vi "config.vi"() -> ()   [LabVIEW 2015]
uses:
  board.vis/Globals.vi
  board.vis/ESLSCDLL.lvlib
panel:
  in  "DLL path select":enum32{"default location", "custom location"}(radio)
  in  "DLL custom path":path
  in  "shift S1S2 to next scan":bool
  in  "channel select":enum32{"Channel A", "Channel B", "Channel A&B"}(ring)=enum."Channel A&B"
  in  "show shutter":bool
  in  "bticnt":u32
  in  "is fft legacy":bool
  in  "s1s2_read_delay_in_10ns":u32
  in  "bnc_out":T1(ring)
  in  "sensor reset or HSIR EC":u32
  in  "SENSOR TYPE":T2(ring)=enum."HSVIS"
  in  "dac":u32[][][](array[numeric])=[[[55000, 52000, 55000, 55000, 55000, 55000, 55000, 55000], [55000, 52000, 55000, 55000, 55000, 55000, 55000, 55000], [55000, 52000, 55000, 55000, 55000, 55000, 55000, 55000], [55000, 52000, 55000, 55000, 55000, 55000, 55000, 55000], [55000, 52000, 55000, 55000, 55000, 55000, 55000, 55000], [55000, 52000, 55000, 55000, 55000, 55000, 55000, 55000], [55000, 52000, 55000, 55000, 55000, 55000, 55000, 55000], [55000, 52000, 55000, 55001, 55000, 55000, 55000, 55000], [55000, 55000, 55000, 55000, 55000, 55000, 55000, 55000], [55000, 55000, 55000, 55000, 55000, 55000, 55000, 55000], [55000, 55000, 55000, 55000, 55000, 55000, 55000, 55000], [55000, 55000, 55000, 55000, 55000, 55000, 55000, 55000]], [[52000, 0, 0, 0, 0, 0, 0, 0], [52000, 0, 0, 0, 0, 0, 0, 0], [52000, 0, 0, 0, 0, 0, 0, 0], [52000, 0, 0, 0, 0, 0, 0, 0], [52000, 0, 0, 0, 0, 0, 0, 0], [52000, 0, 0, 0, 0, 0, 0, 0], [52000, 0, 0, 0, 0, 0, 0, 0], [52000, 0, 0, 0, 0, 0, 0, 0], [0, 0, 0, 0, 0, 0, 0, 0], [0, 0, 0, 0, 0, 0, 0, 0], [0, 0, 0, 0, 0, 0, 0, 0], [0, 0, 0, 0, 0, 0, 0, 0]], [[52000, 0, 0, 0, 0, 0, 0, 0], [52000, 0, 0, 0, 0, 0, 0, 0], [52000, 0, 0, 0, 0, 0, 0, 0], [52000, 0, 0, 0, 0, 0, 0, 0], [52000, 0, 0, 0, 0, 0, 0, 0], [52000, 0, 0, 0, 0, 0, 0, 0], [52000, 0, 0, 0, 0, 0, 0, 0], [52000, 0, 0, 0, 0, 0, 0, 0], [0, 0, 0, 0, 0, 0, 0, 0], [0, 0, 0, 0, 0, 0, 0, 0], [0, 0, 0, 0, 0, 0, 0, 0], [0, 0, 0, 0, 0, 0, 0, 0]], [[52000, 0, 0, 0, 0, 0, 0, 0], [52000, 0, 0, 0, 0, 0, 0, 0], [52000, 0, 0, 0, 0, 0, 0, 0], [52000, 0, 0, 0, 0, 0, 0, 0], [52000, 0, 0, 0, 0, 0, 0, 0], [52000, 0, 0, 0, 0, 0, 0, 0], [52000, 0, 0, 0, 0, 0, 0, 0], [52000, 0, 0, 0, 0, 0, 0, 0], [0, 0, 0, 0, 0, 0, 0, 0], [0, 0, 0, 0, 0, 0, 0, 0], [0, 0, 0, 0, 0, 0, 0, 0], [0, 0, 0, 0, 0, 0, 0, 0]], [[52000, 0, 0, 0, 0, 0, 0, 0], [52000, 0, 0, 0, 0, 0, 0, 0], [52000, 0, 0, 0, 0, 0, 0, 0], [52000, 0, 0, 0, 0, 0, 0, 0], [52000, 0, 0, 0, 0, 0, 0, 0], [52000, 0, 0, 0, 0, 0, 0, 0], [52000, 0, 0, 0, 0, 0, 0, 0], [52000, 0, 0, 0, 0, 0, 0, 0], [0, 0, 0, 0, 0, 0, 0, 0], [0, 0, 0, 0, 0, 0, 0, 0], [0, 0, 0, 0, 0, 0, 0, 0], [0, 0, 0, 0, 0, 0, 0, 0]]]
  in  "stime[ms]":dbl=0.01 format="%-3.3f"
  in  "btime[ms]":dbl=31.0 format="%1.3f"
  in  "sdat in 10ns":u32
  in  "bdat in 10ns":u32
  in  "bti":T3(ring)=enum."BTimer"
  in  "sti":T4(ring)=enum."STimer"
  in  "trigger mode integrator":enum32{"XCK", "Ext. Trig.", "DAT"}(ring)
  in  "bt slope":enum32{"neg", "pos", "both"}(ring)=enum."pos"
  in  "st slope":enum32{"pos", "neg", "both"}(ring)
  in  "custom pattern":u32=100
  in  "adc mode":enum32{"normal", "ramp", "custom pattern"}(ring)
  in  "fft mode":T5(ring)
  in  "cool level":u32
  in  "board_sel":u32=1 format="%05b"
  in  "sticnt":u32
  in  "show pulse gen":bool
  in  "show special pixels":bool
  in  "debug mode":bool
  in  "show one pixel graph":bool
  in  "adc gain":u32
  in  "area lines binning":u32=1
  in  "nor":u32=3
  in  "region size":u32[](array[numeric])=[4, 62, 4, 28, 14, 0, 0, 0]
  in  "LINES":u32=128
  in  "VFREQ":u32=7
  in  "software polling":bool
  in  "led off":bool
  in  "tocnt":u32
  in  "ioctrl impact start pixel":u32=1050
  in  "cont pause in microseconds":u32
  in  "tor":T6(ring)
  in  "write to disc":bool
  in  "file path":path
  in  "cooled camera legacy mode":bool
  in  "cooled cam":bool
  in  "sensor gain":u32
  in  "gpx offset":u32=1000
  in  "xckdly in 10ns (legacy)":u32
  in  "bec in 10\nns":u32
  in  "sec in 10ns":u32
  in  "CAMCNT 4":u32=1
  in  "CAMCNT 3":u32=1
  in  "CAMCNT 2":u32=1
  in  "CAMCNT 1":u32=1
  in  "CAMCNT 0":u32=1
  in  "CAMERA SYSTEM":enum32{"3001", "3010", "3030"}(ring)=enum."3030"
  in  "PIXEL":u32=1024
  # "camera system settings"
  # "measurement settings"
  # "Pixel sizes:\n192\n320\n576\n1024(HSVIS)\n1088\n2112\n4160\n8256"
  # "output PCIe board"
  # "scan exposue control"
  # "pause for continuous mode in µs"
  # "block exposure control"
  # "block delay after trigger"
  # "CAMCNT\nnumber of \ncameras per board"
  # "only for TDC option"
  # "depending on SENSOR TYPE\nthe actual time is\nHSVIS: time = x * 4 ns\nHSIR: time = x * 160 ns"
  # "fft setttings"
  # "only for FL30XX_simple.vi"
  # "labview"
  # "Select boards bitwise. Bit 0 - board 0 ....\nFor one board: 00001"
  # "lines of camera"
  # "Choose how many lines are binned in area mode.\nare_lines_binning should devide lines without remainder"
  # "number of regions for regions of interest mode\n(choose from 2 to 5)"
  # "count of lines for each region.\nWhen 0 is selected for the first region,\nthe lines are equally distributed over all regions.\nWhen selecting custom values,\nthe sum of all regions should equal lines."
  # "High Speed, 3030"
  # "camera 4"
  # "camera 6"
  # "camera 7"
  # "camera 0"
  # "camera 1"
  # "camera 3"
  # "camera 5"
  # "camera 2"
  # "PCIe board (0 ... 4) -->"
  # "channel 0"
  # "keep 0 -->"
  # "channel 1"
  # "keep 0 -->"
  # "channel 2"
  # "channel 3"
  # "channel 4"
  # "channel 5"
  # "channel 6"
  # "channel 7"
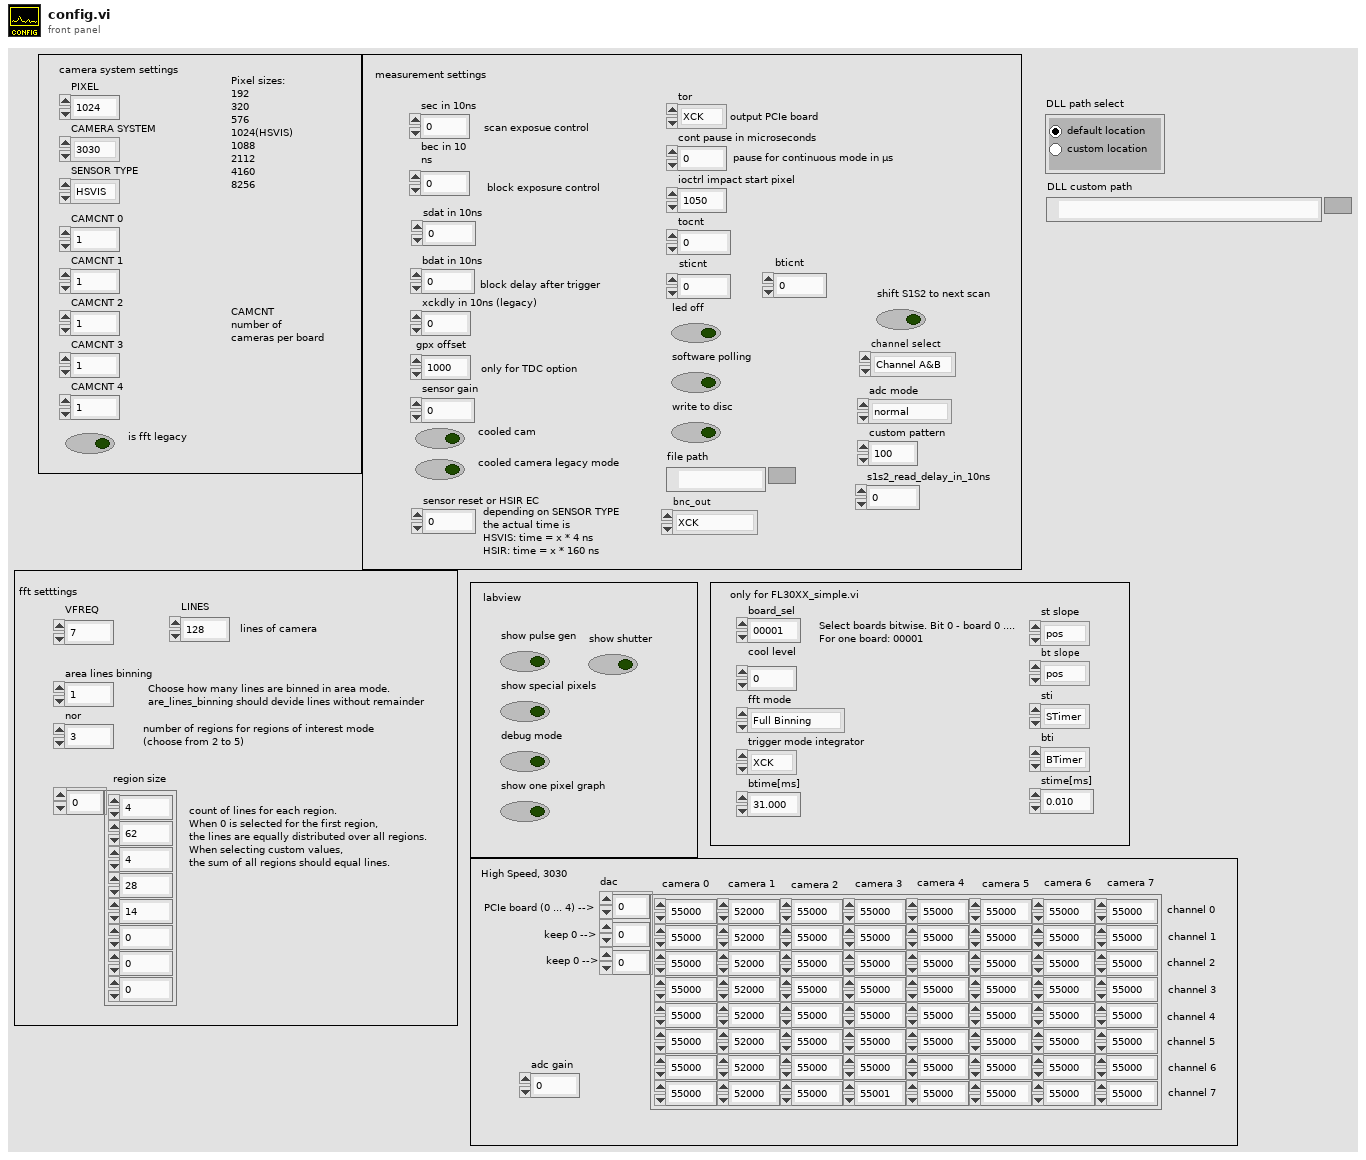
[diagram p1: front panel]
types:
  T1 = enum32{"XCK", "EXP_WIN", "ADC_CLK", "Vin sample"}
  T2 = enum32{"PDA", "IR", "FFT", "CMOS", "HSVIS", "HSIR"}
  T3 = enum32{"I", "S1", "S2", "S1&S2", "BTimer", "S1 chopper", "S2 chopper", "S1&S2 chopper"}
  T4 = enum32{"I", "S1", "S2", "S2=EN_I", "STimer", "ASL"}
  T5 = enum32{"Full Binning", "Region of Interest", "Area"}
  T6 = enum32{"XCK", "Reg/OutTrig", "VON", "DMA_Act", "ASLS", "STIMER", "BTIMER", "INTRSR", "S1", "S2", "BLOCK_ON_SYNCED", "MEASUREON", "SDAT", "BDAT", "SSHUT", "BSHUT", "IFC", "DO_CC_I", "EXPOSURE_WINDOW", "TO_CNT_OUT", "SECON", "I", "S1S2ReadDelay", "BLOCK_ON", "unused4", "unused5", "unused6", "unused7", "unused8", "ENFFR", "ENFFW", "ENFFWRPROT"}
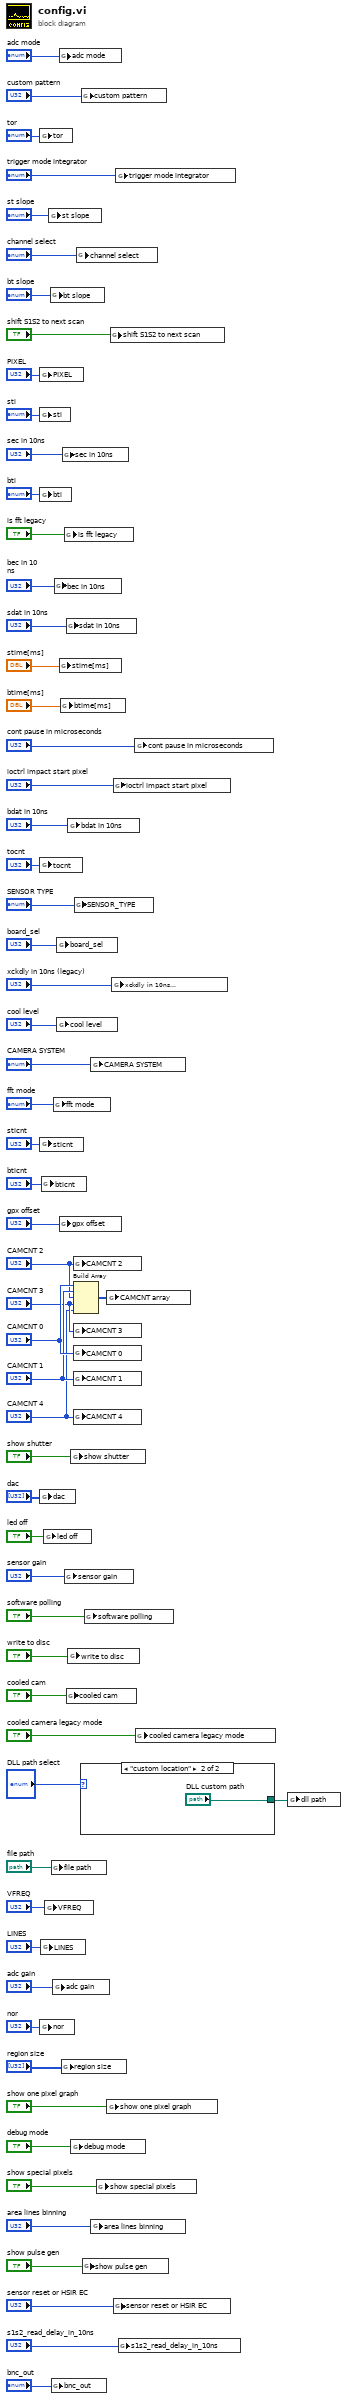
[diagram p0: block diagram]
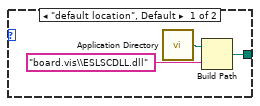
[diagram p2: hidden frame]
diagram:
  n1 = global write "Globals.vi" "tor"("tor") -> ()
  n2 = global write "Globals.vi" "PIXEL"("PIXEL") -> ()
  n3 = global write "Globals.vi" "sti"("sti") -> ()
  n4 = global write "Globals.vi" "bti"("bti") -> ()
  n5 = global write "Globals.vi" "tocnt"("tocnt") -> ()
  n6 = global write "Globals.vi" "sticnt"("sticnt") -> ()
  n7 = global write "Globals.vi" "dac"("dac") -> ()
  n8 = global write "Globals.vi" "nor"("nor") -> ()
  n9 = global write "Globals.vi" "LINES"("LINES") -> ()
  n10 = global write "Globals.vi" "bticnt"("bticnt") -> ()
  n11 = global write "Globals.vi" "led off"("led off") -> ()
  n12 = global write "Globals.vi" "VFREQ"("VFREQ") -> ()
  n13 = global write "Globals.vi" "st slope"("st slope") -> ()
  n14 = global write "Globals.vi" "bt slope"("bt slope") -> ()
  n15 = global write "Globals.vi" "file path"("file path") -> ()
  n16 = global write "Globals.vi" "bnc_out"("bnc_out") -> ()
  n17 = global write "Globals.vi" "adc gain"("adc gain") -> ()
  n18 = global write "Globals.vi" "fft mode"("fft mode") -> ()
  n19 = global write "Globals.vi" "bec in 10ns"("bec in 10\nns") -> ()
  n20 = global write "Globals.vi" "board_sel"("board_sel") -> ()
  n21 = global write "Globals.vi" "cool level"("cool level") -> ()
  n22 = global write "Globals.vi" "adc mode"("adc mode") -> ()
  n23 = global write "Globals.vi" "stime[ms]"("stime[ms]") -> ()
  n24 = global write "Globals.vi" "gpx offset"("gpx offset") -> ()
  n25 = global write "Globals.vi" "btime[ms]"("btime[ms]") -> ()
  n26 = global write "Globals.vi" "region size"("region size") -> ()
  n27 = global write "Globals.vi" "sec in 10ns"("sec in 10ns") -> ()
  n28 = global write "Globals.vi" "is fft legacy"("is fft legacy") -> ()
  n29 = global write "Globals.vi" "sensor gain"("sensor gain") -> ()
  n30 = global write "Globals.vi" "sdat in 10ns"("sdat in 10ns") -> ()
  n31 = global write "Globals.vi" "cooled cam"("cooled cam") -> ()
  n32 = global write "Globals.vi" "bdat in 10ns"("bdat in 10ns") -> ()
  n33 = global write "Globals.vi" "write to disc"("write to disc") -> ()
  n34 = global write "Globals.vi" "show shutter"("show shutter") -> ()
  n35 = global write "Globals.vi" "debug mode"("debug mode") -> ()
  n36 = global write "Globals.vi" "CAMCNT 2"("CAMCNT 2") -> ()
  n37 = Build Array("CAMCNT 0", "CAMCNT 1", "CAMCNT 2", "CAMCNT 3", "CAMCNT 4") -> (w55:u32[])
  n38 = global write "Globals.vi" "CAMCNT 3"("CAMCNT 3") -> ()
  n39 = global write "Globals.vi" "CAMCNT 0"("CAMCNT 0") -> ()
  n40 = global write "Globals.vi" "CAMCNT 1"("CAMCNT 1") -> ()
  n41 = global write "Globals.vi" "CAMCNT 4"("CAMCNT 4") -> ()
  n42 = global write "Globals.vi" "SENSOR_TYPE"("SENSOR TYPE") -> ()
  n43 = global write "Globals.vi" "channel select"("channel select") -> ()
  n44 = case shown="\"custom location\"" "DLL path select" {
    tunnel: [w61 "DLL custom path"] -> w1
    frame "default location", Default {
      n45 = call <vilib>:"Application Directory.vi"() -> ("Application Directory"=w62:path)
      n46 = Build Path(base path=w62, name or relative path="board.vis\\ESLSCDLL.dll") -> (appended path=w61:path)
    }
    frame "custom location" {
    }
  }
  n47 = global write "Globals.vi" "custom pattern"("custom pattern") -> ()
  n48 = global write "Globals.vi" "show pulse gen"("show pulse gen") -> ()
  n49 = global write "Globals.vi" "software polling"("software polling") -> ()
  n50 = global write "Globals.vi" "CAMERA SYSTEM"("CAMERA SYSTEM") -> ()
  n51 = global write "Globals.vi" "area lines binning"("area lines binning") -> ()
  n52 = global write "Globals.vi" "show special pixels"("show special pixels") -> ()
  n53 = global write "Globals.vi" "CAMCNT array"(w55) -> ()
  n54 = global write "Globals.vi" "show one pixel graph"("show one pixel graph") -> ()
  n55 = global write "Globals.vi" "shift S1S2 to next scan"("shift S1S2 to next scan") -> ()
  n56 = global write "Globals.vi" "xckdly in 10ns\n(legacy)"("xckdly in 10ns (legacy)") -> ()
  n57 = global write "Globals.vi" "ioctrl impact start pixel"("ioctrl impact start pixel") -> ()
  n58 = global write "Globals.vi" "sensor reset or HSIR EC"("sensor reset or HSIR EC") -> ()
  n59 = global write "Globals.vi" "trigger mode integrator"("trigger mode integrator") -> ()
  n60 = global write "Globals.vi" "s1s2_read_delay_in_10ns"("s1s2_read_delay_in_10ns") -> ()
  n61 = global write "Globals.vi" "cont pause in microseconds"("cont pause in microseconds") -> ()
  n62 = global write "Globals.vi" "cooled camera legacy mode"("cooled camera legacy mode") -> ()
  n63 = global write "Globals.vi" "dll path"(w1) -> ()
